vi "Append Carriage Return Character.vi"(8 "error in (no error)":errorcluster, 11 "Command":string) -> (0 "error out":errorcluster, 3 "Command Out":string)   [LabVIEW 2012, in "YOST 3 Space.lvlib"]
uses:
  YOST 3 Space.lvlib
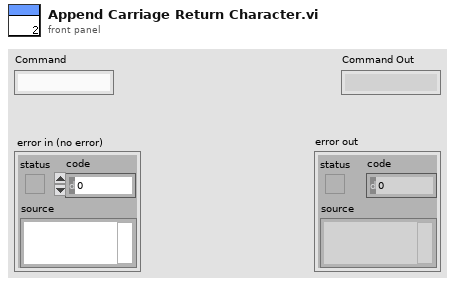
[diagram p1: front panel]
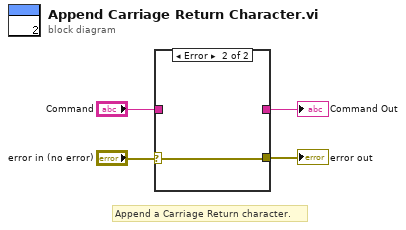
[diagram p0: block diagram]
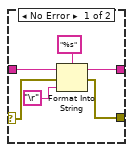
[diagram p2: hidden frame]
diagram:
  # "Append a Carriage Return character."
  n1 = case shown="Error" "error in (no error)" {
    selector: "error in (no error)" -> [w7 w11]
    tunnel: "Command" -> [w10 _]
    tunnel: [w6 _] -> w1
    tunnel: [w5 w11] -> w2
    frame No Error {
      n2 = Format Into String(format string="%s", initial string=w10, error in=w7, "\r") -> (resulting string=w6:string, error out=w5:errorcluster)
    }
    frame Error {
    }
  }
  "Command Out" <- w1
  "error out" <- w2
